vi "ikine.vi"(11 "Tip XYZ Posit [mm]":dbl[](array[numeric])=[0.0, 1.0, 0.0]) -> (3 "Joint Posit [deg,deg,mm]":dbl[](array[numeric])=[0.0, 1.0, 0.0])   [LabVIEW 2016]
doc: "This VI converts the desired tool tip position (px,py,pz) [mm] into joint motions of theta 1, theta 2, and theta 3 [counts]."
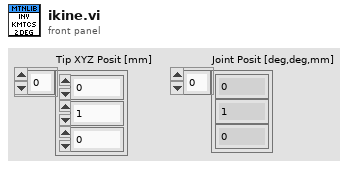
[diagram p1: front panel]
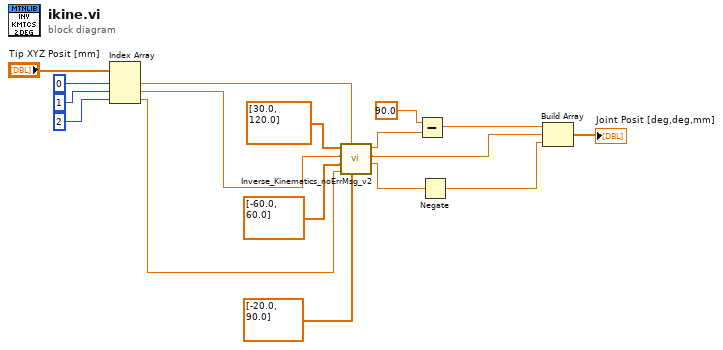
[diagram p0: block diagram]
diagram:
  n1 = Index Array(array="Tip XYZ Posit [mm]", index #1=0 ("index"), index #2=1 ("index"), index #3=2 ("index")) -> (element #1=w10:dbl, element #2=w9:dbl, element #3=w8:dbl)
  n2 = call "Inverse_Kinematics_noErrMsg_v2.vi"("B3"=dbl[] [-20.0, 90.0], "px"=w10, "pz"=w8, "B2"=dbl[] [-60.0, 60.0], "py"=w9, "B1"=dbl[] [30.0, 120.0]) -> ("theta 3"=w13:dbl, "theta 2"=w2:dbl, "theta 1"=w12:dbl)  [unwired: 1 in]
  n3 = Subtract(x=90.0, y=w12) -> (x-y=w3:dbl)
  n4 = Negate(x=w13) -> (-x=w1:dbl)
  n5 = Build Array(w3, w2, w1) -> (→"Joint Posit [deg,deg,mm]":dbl[])
